vi "Select visible data.vi"(11 "Data ref":refnum<vi>) -> (1 "Cursors":dbl[](array[numeric]), 2 "dt":dbl, 3 "Visible Data":dbl[][](array[numeric]))   [LabVIEW 2016]
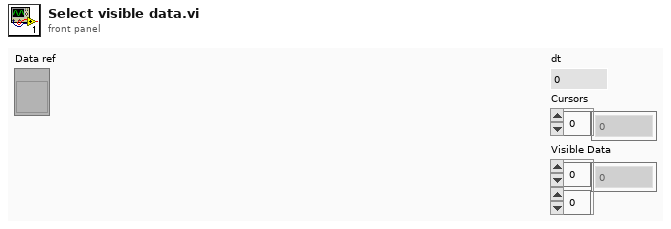
[diagram p1: front panel]
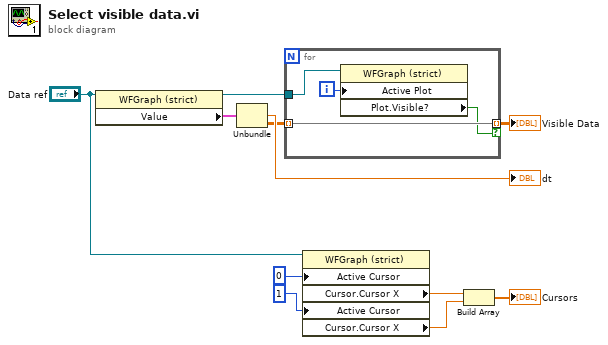
[diagram p0: block diagram]
diagram:
  n1 = property class="WFGraph (strict)"(reference="Data ref") -> (reference out=w3:refnum<vi>, "Value"=w7:cluster{dbl, dbl, "Impulses":dbl[][]})  [unwired: 1 in, 1 out]
  n2 = Unbundle(w7) -> (→"dt":dbl, "Impulses"=w4:dbl[][])  [unwired: 1 out]
  n3 = for {
    tunnel: w4 -> [w13] mode=indexing
    tunnel: w3 -> [w14]
    tunnel: [w13] -> w1 mode=indexing if=w12
    i -> [w15]
    n4 = property class="WFGraph (strict)"(reference=w14, "Active Plot"=w15) -> ("Plot.Visible?"=w12:bool)  [unwired: 1 in, 2 out]
  }
  "Visible Data" <- w1
  n5 = property class="WFGraph (strict)"(reference="Data ref", "Active Cursor"=0, "Active Cursor"=1) -> ("Cursor.Cursor X"=w10:dbl, "Cursor.Cursor X"=w11:dbl)  [unwired: 1 in, 2 out]
  n6 = Build Array(w10, w11) -> (→"Cursors":dbl[])
